vi "Handle Error.vi"(8 "error in (no error)":errorcluster, 11 "Camera Actor in":refnum<class "Camera Actor.lvclass">) -> (0 "error out":errorcluster, 2 "stop actor?":bool=TRUE, 3 "Camera Actor out":refnum<class "Camera Actor.lvclass">)   [LabVIEW 2014, in "Camera Actor.lvlib" / "Camera Actor.lvclass"]
doc: "(<B>Filename</B>: Actor Framework.lvlib:Actor.lvclass:Handle Error.vi)\n\nDefines how the actor handles an error that occurred while processing a message. By default, this method does nothing except stop the actor."
uses:
  Camera Actor.lvclass
  <vilib>/ActorFramework/Actor/Actor.lvclass
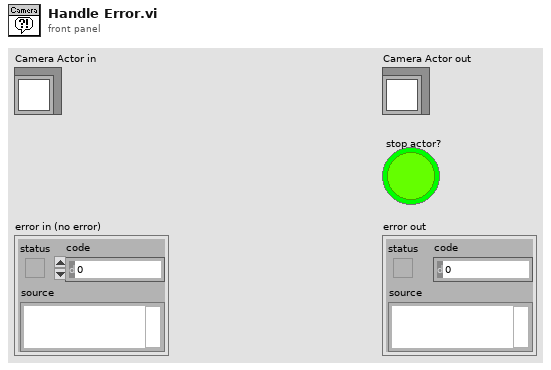
[diagram p1: front panel]
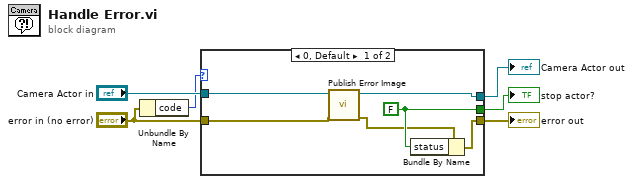
[diagram p0: block diagram]
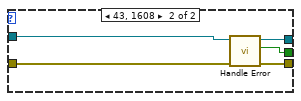
[diagram p2: hidden frame]
diagram:
  n1 = Unbundle By Name("error in (no error)") -> ("code"=w1:i32)
  n2 = case shown="0, Default" w1 {
    tunnel: [w11 w17] -> w6
    tunnel: [w10 w16] -> w5
    tunnel: [w9 w15] -> w4
    tunnel: "error in (no error)" -> [w8 w14]
    tunnel: "Camera Actor in" -> [w12 w13]
    frame 0, Default {
      w10 = FALSE ("status")
      n3 = call-dynamic "Publish Error Image.vi"("error in (no error)"=w8, "Camera Actor in"=w12) -> ("error out"=w7:errorcluster, "Camera Actor out"=w9:refnum<class "Camera Actor.lvclass">)  [unwired: 8 in]
      n4 = Bundle By Name(cluster=w7, "status"=w10) -> (w11:errorcluster)
    }
    frame 43, 1608 {
      n5 = call-parent "Handle Error.vi"("error in (no error)"=w14, "Actor in"=w13) -> ("error out"=w17:errorcluster, "stop actor?"=w16:bool, "Actor out"=w15:refnum<class "Camera Actor.lvclass">)  [unwired: 7 in]
    }
  }
  "Camera Actor out" <- w4
  "error out" <- w6
  "stop actor?" <- w5
